vi "Drive Encoder Counter.vi"   [LabVIEW 2010]
uses:
  Motor Encoder Global.vi
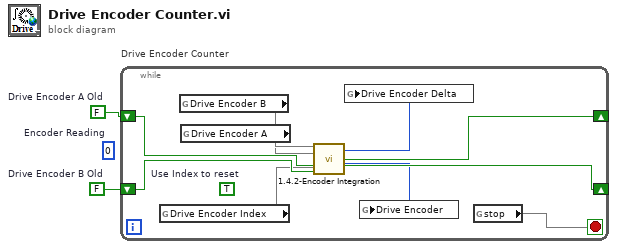
[diagram p0: block diagram]
diagram:
  (unwired) 0  # Encoder Reading
  w2 = FALSE  # Drive Encoder A Old
  w1 = FALSE  # Drive Encoder B Old
  n1 = while "Drive Encoder Counter" {
    shift-right: [w12] -> _
    shift-left: w2 -> [w11]
    shift-right: [w10] -> _
    shift-left: w1 -> [w9]
    stop <- w8 stop-if-true
    (unwired) TRUE  # Use Index to reset
    n2 = global read "Motor Encoder Global.vi" "Drive Encoder Index"() -> (w5)
    n3 = global read "Motor Encoder Global.vi" "Drive Encoder B"() -> (w7)
    n4 = global read "Motor Encoder Global.vi" "Drive Encoder A"() -> (w6)
    n5 = call "1.4.2-Encoder Integration.vi"("Encoder B"=w7, "Encoder A"=w6, "Encoder A Old"=w11, "Encoder B Old"=w9, "Encoder Index"=w5) -> ("Count Delta"=w3:i32, "Encoder A Old (sReg)"=w12:bool, "Encoder B Old (sReg)"=w10:bool, "Current count"=w4:i32)  [unwired: 5 in, 2 out]
    n6 = global write "Motor Encoder Global.vi" "Drive Encoder Delta"(w3) -> ()
    n7 = global write "Motor Encoder Global.vi" "Drive Encoder"(w4) -> ()
    n8 = global read "Motor Encoder Global.vi" "stop"() -> (w8)
  }
